vi "UsrProfiles-Update users list.vi"(8 "error in":errorcluster) -> (0 "error out":errorcluster)   [LabVIEW 2013]
uses:
  Globals/gl_UsrProfiles globals.vi
  Global Variables/General Globals.vi
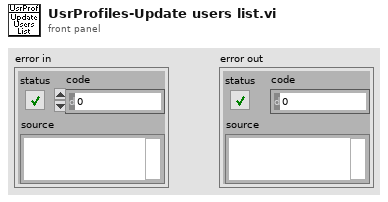
[diagram p1: front panel]
types:
  T1 = typedef "User login window refs.ctl" = cluster{"User profiles window ref":refnum<k9>, "Users listbox":refnum<vi>, "Profiles listbox":refnum<vi>, "Last used":refnum<vi>}
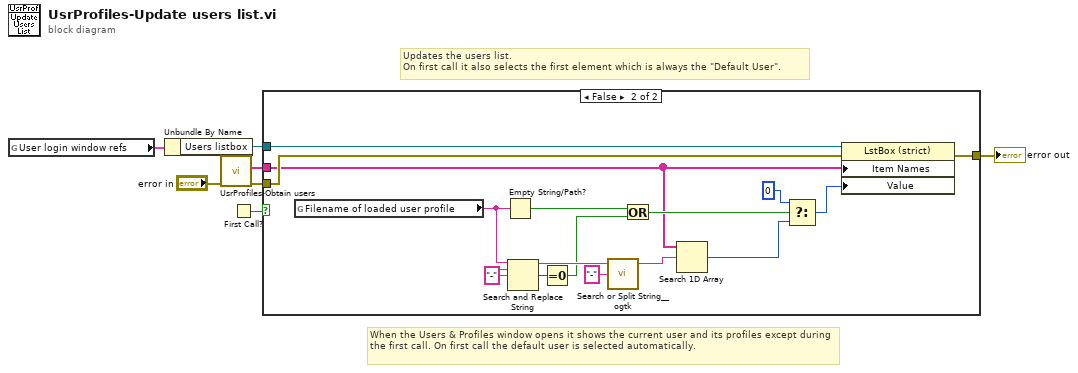
[diagram p0: block diagram]
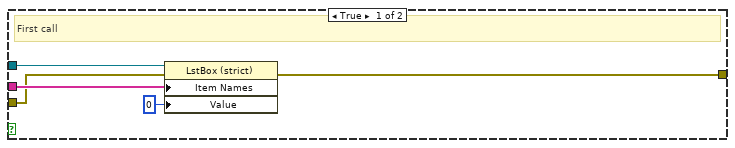
[diagram p2: hidden frame]
diagram:
  # "When the Users & Profiles window opens it shows the current user and its profiles except during the first call. On first call the default user is selected automatically."
  # "Updates the users list.\nOn first call it also selects the first element which is always the \"Default User\"."
  n1 = global read "gl_UsrProfiles globals.vi" "User login window refs"() -> (w6:T1)
  n2 = Unbundle By Name(w6) -> ("Users listbox"=w7:refnum<vi>)
  n3 = call "UsrProfiles-Obtain users.vi"("error in"="error in") -> ("error out"=w5:errorcluster, "User names"=w2:string[])  [unwired: 9 in]
  n4 = First Call?() -> (First Call?: T/F=w1:bool)
  n5 = case shown="False" w1 {
    tunnel: w2 -> [w12 w13]
    tunnel: w7 -> [w11 w28]
    tunnel: [w9 w27] -> w3
    tunnel: w5 -> [w8 w26]
    frame True {
      # "First call"
      n6 = property on="Property Node" class="LstBox (strict)"(reference=w11, error in=w8, "Item Names"=w12, "Value"=0) -> (error out=w9:errorcluster)  [unwired: 1 out]
    }
    frame False {
      w17 = "-" ("search string/char (-)")
      n7 = global read "General Globals.vi" "Filename of loaded user profile"() -> (w16:string)
      n8 = Empty String/Path?(string/path=w16) -> (empty?=w19:bool)
      n9 = Search and Replace String(input string=w16, search string=w17, replace string=w17) -> (result string=w22:string, number of replacements=w18:i32)  [unwired: 5 in, 2 out]
      n10 = Equal To 0?(x=w18) -> (x = 0?=w21:bool)
      n11 = call "Search or Split String__ogtk.vi"("search string/char (-)"="-", "string"=w22) -> ("substring before match"=w24:string)  [unwired: 1 in, 2 out]
      n12 = Or(x=w19, y=w21) -> (x .or. y?=w20:bool)
      n13 = Search 1D Array(1D array=w13, element=w24) -> (index of element=w25:i32)  [unwired: 1 in]
      n14 = Select(t=0 ("Value"), s=w20, f=w25) -> (s? t:f=w15:i32)
      n15 = property on="Property Node" class="LstBox (strict)"(reference=w28, error in=w26, "Item Names"=w13, "Value"=w15) -> (error out=w27:errorcluster)  [unwired: 1 out]
    }
  }
  "error out" <- w3
